vi "Newmark-CorrectPosition.vi"(0 "Table VRN IN":refnum<visa-resource-name>, 2 "Bool Refnum":refnum<vi>, 11 "Error IN":errorcluster, 12 "StageTags":string[](array[string]), 13 "Corrections":dbl[](array[numeric])) -> (4 "Table VRN OUT":refnum<visa-resource-name>, 8 "Erreur":bool, 15 "Error OUT":errorcluster)   [LabVIEW 2019]
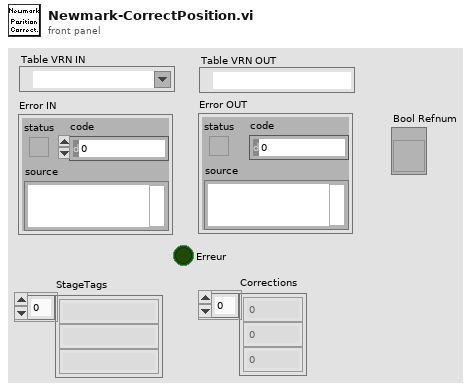
[diagram p1: front panel]
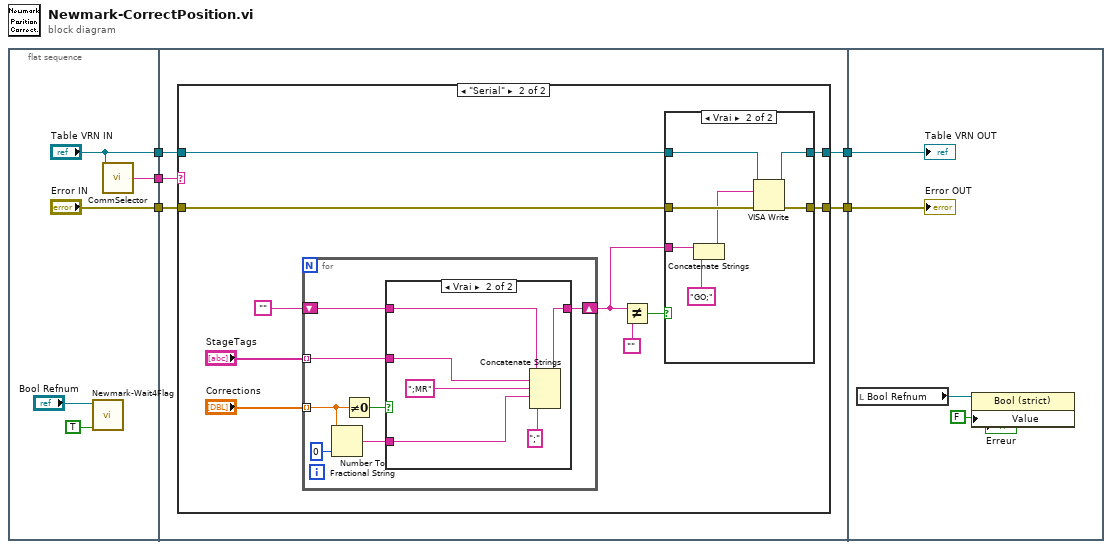
[diagram p0: block diagram]
diagram:
  n1 = flat-sequence {
    tunnel: [w8] -> w5
    tunnel: ["Error IN"] -> w4
    tunnel: ["Table VRN IN"] -> w3
    tunnel: w3 -> [w13]
    tunnel: w4 -> [w14]
    tunnel: w5 -> [w15]
    tunnel: [w12] -> w2
    tunnel: [w11] -> w1
    tunnel: w2 -> [w51]
    tunnel: w1 -> [w52]
    frame #0 {
      n2 = call "Newmark-Wait4Flag.vi"("Raise Flag ?"=TRUE, "Ctl Refnum IN"="Bool Refnum") -> ()  [unwired: 8 in, 2 out]
      n3 = call "CommSelector.vi"("VISA resource name"="Table VRN IN") -> ("CommType"=w8:string)  [unwired: 13 in, 1 out]
    }
    frame #1 {
      n4 = case shown="\"Serial\"" w15 {
        tunnel: w14 -> [w16 w22]
        tunnel: w13 -> [w17 w23]
        tunnel: [w16 w21] -> w12
        tunnel: [w17 w20] -> w11
        frame "Unknown", Default {
        }
        frame "Serial" {
          n5 = for {
            tunnel: "Corrections" -> [w41] mode=indexing
            shift-right: [w38] -> w24
            shift-left: "" -> [w42]
            tunnel: "StageTags" -> [w37] mode=indexing
            n6 = Number To Fractional String(number=w41, precision (6)=i16 0) -> (F-format string=w40:string)  [unwired: 2 in]
            n7 = Not Equal To 0?(x=w41) -> (x != 0?=w43:bool)
            n8 = case shown="Vrai" w43 {
              tunnel: w42 -> [w44 w46]
              tunnel: w40 -> [_ w50]
              tunnel: [w44 w49] -> w38
              tunnel: w37 -> [_ w45]
              frame False {
              }
              frame True {
                n9 = Concatenate Strings(w46, w45, ";MR", w50, ";" ("string")) -> (w49:string)
              }
            }
          }
          n10 = Not Equal?(x=w24, y="") -> (x != y?=w25:bool)
          n11 = case shown="Vrai" w25 {
            tunnel: w24 -> [_ w32]
            tunnel: w23 -> [w29 w35]
            tunnel: w22 -> [w28 w36]
            tunnel: [w29 w34] -> w20
            tunnel: [w28 w33] -> w21
            frame False {
            }
            frame True {
              n12 = Concatenate Strings(w32, "GO;") -> (w30:string)
              n13 = VISA Write(VISA resource name=w35, write buffer=w30, error in (no error)=w36) -> (VISA resource name out=w34:refnum<visa-resource-name>, error out=w33:errorcluster)  [unwired: 1 out]
            }
          }
        }
      }
    }
    frame #2 {
      n14 = local read "Bool Refnum"() -> (w54:refnum<vi>)
      n15 = property class="Bool (strict)"(reference=w54, "Value"=FALSE) -> ()  [unwired: 1 in, 2 out]
      "Table VRN OUT" <- w52
      "Error OUT" <- w51
    }
  }
